vi "Compute Next Cron.vi"(6 "Ignore DST?":bool, 8 "error in (no error)":errorcluster, 10 "Time Stamp (Now)":timestamp, 11 "Cron in":refnum<class "Cron.lvclass">) -> (0 "error out":errorcluster, 1 "Occurence found":bool, 2 "Next Occurence":timestamp, 3 "Cron out":refnum<class "Cron.lvclass">)   [LabVIEW 2013, in "openCron.lvlib" / "Cron.lvclass"]
doc: "Set the \"Ignore DST\" flag to true if you want the timestamp to not take daylight saving time transitions into account when computing the next cron time. This is useful for displaying the future cron job timestamps when the query is made at a time during DST but the result is outside DST period. The timestamp would display a 1-hour discrepency during that period if the flag is false. This is normal and consistent because the local system will adjust this 1-hour difference when the DST change date is crossed.\n\nFor planning purposes, the flag should stay False.\nFor printing a list of future cron jobs time, it is useful to ignore the DST changes, so the flag should be set True."
uses:
  Cron.lvclass
  Cron.lvclass/Cron.ctl
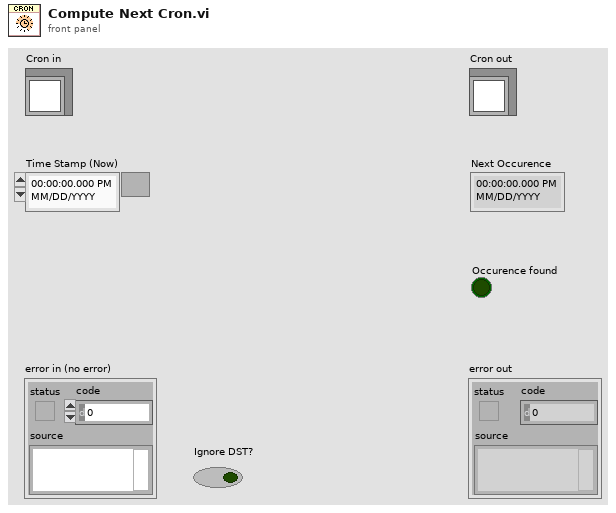
[diagram p1: front panel]
types:
  T1 = typedef "openCron.lvlib/Cron.lvclass/CronTime -- cluster.ctl" = cluster{"second":i32, "minute":i32, "hour":i32, "day of month":i32, "month":i32, "day of week":i32, "year":i32}
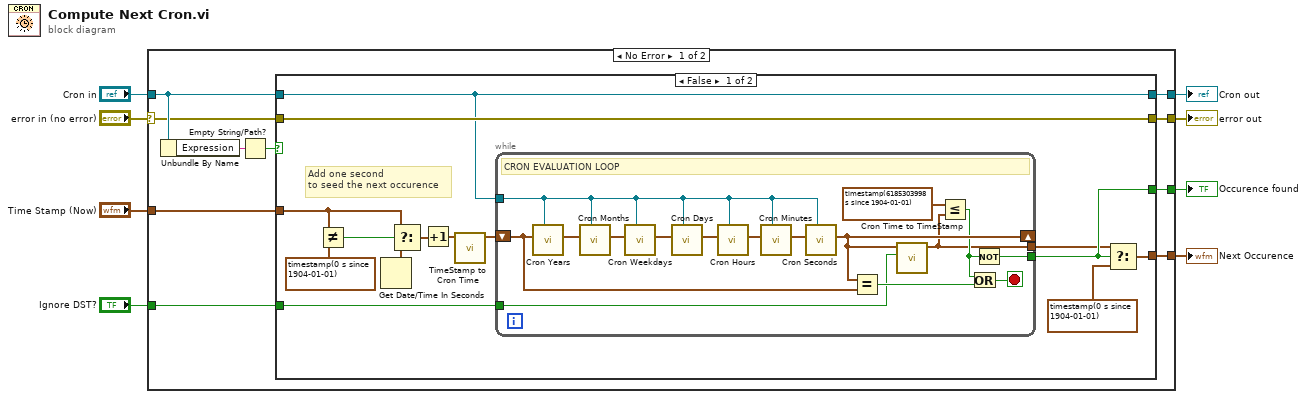
[diagram p0: block diagram]
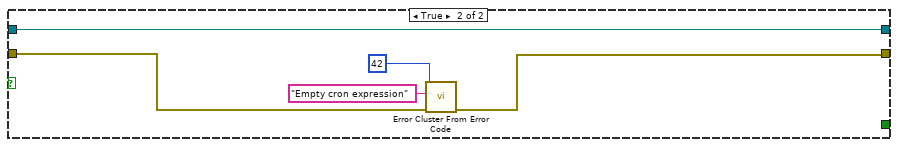
[diagram p2: hidden frame]
diagram:
  n1 = case shown="No Error" "error in (no error)" {
    selector: "error in (no error)" -> [w12 w54]
    tunnel: [w11 w54] -> w7
    tunnel: [w10 w55] -> w5
    tunnel: "Cron in" -> [w15 w55]
    tunnel: "Time Stamp (Now)" -> [w18 _]
    tunnel: [w17 _] -> w2
    tunnel: [w16 _] -> w3
    tunnel: "Ignore DST?" -> [w9 _]
    frame No Error {
      n2 = Unbundle By Name(w15) -> ("Expression"=w14:string)
      n3 = Empty String/Path?(string/path=w14) -> (empty?=w13:bool)
      n4 = case shown="False" w13 {
        tunnel: w18 -> [w30 _]
        tunnel: [w24 _] -> w17
        tunnel: [w23 _] -> w16
        tunnel: w15 -> [w26 w53]
        tunnel: w12 -> [w27 w51]
        tunnel: [w27 w52] -> w11
        tunnel: [w26 w53] -> w10
        tunnel: w9 -> [w19 _]
        frame False {
          # "Add one second\nto seed the next occurence"
          n5 = Not Equal?(x=w30, y=timestamp(0 s since 1904-01-01)) -> (x != y?=w31:bool)
          n6 = Get Date/Time In Seconds() -> (seconds since 1Jan1904=w29:timestamp)
          n7 = Select(t=w30, s=w31, f=w29) -> (s? t:f=w21:timestamp)
          n8 = Increment(x=w21) -> (x+1=w20:timestamp)
          n9 = call "TimeStamp to Cron Time.vi"("Time Stamp"=w20) -> ("Cron Time"=w28:T1)  [unwired: 10 in]
          n10 = while {
            shift-right: [w37] -> _
            shift-left: w28 -> [w45]
            tunnel: w26 -> [w44]
            tunnel: [w35] -> w23
            tunnel: [w34] -> w22
            tunnel: w19 -> [w33]
            stop <- w41 stop-if-true
            # "CRON EVALUATION LOOP"
            n11 = call "Cron Years.vi"(7:"Cron"=w44, 10:"Cron"=w45) -> ("Cron Time"=w48:T1)  [unwired: 9 in]
            n12 = call "Cron Months.vi"(7:"Cron"=w44, 10:"Cron"=w48) -> ("Cron Time"=w40:T1)  [unwired: 9 in]
            n13 = call "Cron Weekdays.vi"(7:"Cron"=w44, 10:"Cron"=w40) -> ("Cron Time"=w39:T1)  [unwired: 9 in]
            n14 = call "Cron Days.vi"(7:"Cron"=w44, 10:"Cron"=w39) -> ("Cron Time"=w38:T1)  [unwired: 9 in]
            n15 = call "Cron Hours.vi"(7:"Cron"=w44, 10:"Cron"=w38) -> ("Cron Time"=w47:T1)  [unwired: 9 in]
            n16 = call "Cron Minutes.vi"(7:"Cron"=w44, 10:"Cron"=w47) -> ("Cron Time"=w46:T1)  [unwired: 9 in]
            n17 = call "Cron Seconds.vi"(7:"Cron"=w44, 10:"Cron"=w46) -> ("Cron Time"=w37:T1)  [unwired: 9 in]
            n18 = Equal?(x=w37, y=w45) -> (x = y?=w42:bool)
            n19 = call "Cron Time to TimeStamp.vi"("Correct for DST?"=w33, "Cron Time"=w37) -> ("Time Stamp"=w34:timestamp)  [unwired: 9 in]
            n20 = Less Or Equal?(x=timestamp(6185303998 s since 1904-01-01) ("y"), y=w34) -> (x <= y?=w36:bool)
            n21 = Or(x=w36, y=w42) -> (x .or. y?=w41:bool)
            n22 = Not(x=w36) -> (.not. x?=w35:bool)
          }
          n23 = Select(t=w22, s=w23, f=timestamp(0 s since 1904-01-01) ("y")) -> (s? t:f=w24:timestamp)
        }
        frame True {
          n24 = call <vilib>:"Error Cluster From Error Code.vi"("error in (no error)"=w51, "error message (\"\")"="Empty cron expression" ("error message (\"\")"), "error code (0)"=42) -> ("error out"=w52:errorcluster)  [unwired: 6 in]
        }
      }
    }
    frame Error {
    }
  }
  "error out" <- w7
  "Cron out" <- w5
  "Next Occurence" <- w2
  "Occurence found" <- w3
